vi "VI Server_Get Control_Value_StringFormat.vi"(7 "Label":string, 8 "error in (no error)":errorcluster, 11 "VI Server Cluster":T1) -> (0 "error out":errorcluster, 1 "ControlValue(StringFormat)":string, 2 "FloatingData":bool, 3 "VI Server Cluster.DUP":T1)   [LabVIEW 2020, in "VI Server Toolkit LV2013.lvlib"]
doc: "Returns control's value formatted as string.\nUsed for saving such values into configuration file."
uses:
  VI Server Toolkit LV2013.lvlib
  VI Server_TypeDefs/VI Server_RefsCluster.ctl
  VI Server Libraries/VI Server Controls.llb/VI Server_GetSet Controls From String Format_Options.ctl
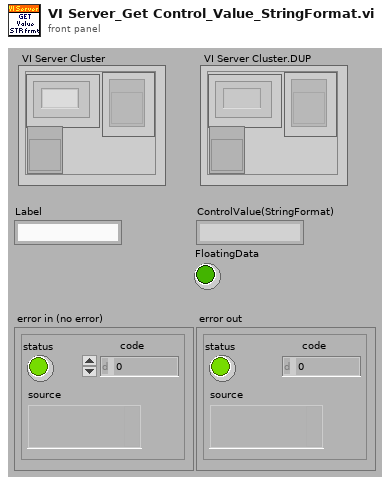
[diagram p1: front panel]
types:
  T1 = typedef "VI Server_RefsCluster.ctl" = cluster{"Labels":string[], "Refs":refnum<vi>[], "VI Ref":refnum<vi>}
  T2 = typedef "VI Server Toolkit LV2013.lvlib/VI Server_GetSet Controls From String Format_Options.ctl" = enum16{"", "If Ring Get Selection", "If Ring Set by Selection"}
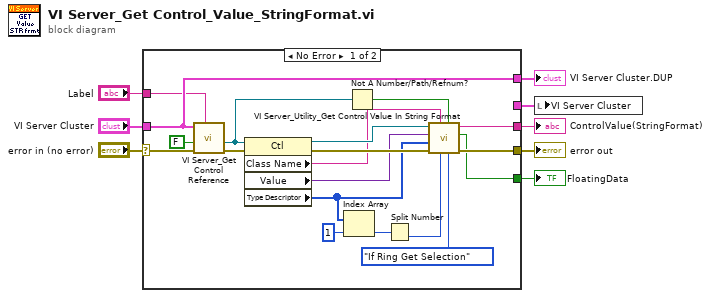
[diagram p0: block diagram]
diagram:
  n1 = case shown="No Error" "error in (no error)" {
    selector: "error in (no error)" -> [w25 w29]
    tunnel: [w18 w29] -> w8
    tunnel: "VI Server Cluster" -> [w23 _]
    tunnel: "Label" -> [w22 _]
    tunnel: [w11 _] -> w4
    tunnel: [w23 _] -> w3
    tunnel: [_ w28] -> w2
    tunnel: [w9 _] -> w1
    frame No Error {
      n2 = call "VI Server_Get Control Reference.vi"("Label"=w22, "error in"=w25, "Single Instance (T)"=FALSE, "VI Server Cluster"=w23) -> ("error out"=w24:errorcluster, "Control Reference (Generic)"=w21:refnum<vi>)  [unwired: 4 in, 2 out]
      n3 = property class="Ctl"(reference=w21, error in=w24) -> (reference out=w17:refnum<vi>, error out=w19:errorcluster, "Class Name"=w15:string, "Value"=w14:variant, "Type Descriptor"=w12:i16[])
      n4 = Index Array(array=w12, index=1) -> (element=w26:i16)
      n5 = Not A Number/Path/Refnum?(number/path/refnum=w21) -> (NaN/Path/Refnum?=w16:bool)
      n6 = Split Number(x=w26) -> (lo(x)=w13:u8)  [unwired: 1 out]
      n7 = call "VI Server_Utility_Get Control Value In String Format.vi"("Options"=VI_Server_GetSet_Controls_From_String_Format_Options."If Ring Get Selection", "Continue"=w16, "Control.Representation"=w13, "Control.ClassName"=w15, "error in (no error)"=w19, "TypeDesc"=w12, "Control.Value.Invariant"=w14, "Control.Ref"=w17) -> ("error out"=w18:errorcluster, "FloatingData"=w9:bool, "Control.String.OUT"=w11:string)  [unwired: 1 out]
    }
    frame Error {
      n8 = call "VI Server_Empty VI Server Cluster.vi"() -> ("VI Server Cluster"=w28:T1)  [unwired: 7 in]
    }
  }
  "error out" <- w8
  "VI Server Cluster.DUP" <- w3
  "ControlValue(StringFormat)" <- w4
  "FloatingData" <- w1
  n9 = local write "VI Server Cluster"(w2) -> ()
